vi "re_do_task_lua.vi"(5 "LuaVIEW reference":T1) -> (15 "error out":errorcluster)   [LabVIEW 2012]
doc: "Call the \"Do Task\" Lua API VI to prepare, pre-process, and execute a task script. Though this creates a seperate execution context, this function is synchronous because it waits for the task to finish.\n\nBy calling this function through <code>lv.pcall()</code>, you can execute, in a task context, a bit of code that can throw errors or has other ill-defined behaviour without risking the termination of your script or the corruption of its variable space.\n\nIf the task script is contained in a file, a relative path or bare filename will be resolved by searching relative to the configured script search directories. If no script search directories are configured, the resource base path is searched. If this function is called from a task context, the directory holding the main script of the calling task is searched first.\nParameters:\nstr:name, when the optional task script string is not specified, this is the filename plus any path from which to load the task script. Otherwise it is the name used to refer to the task script when reporting errors.\n[str:script], optional task script string allows direct specification of a bit of Lua code.\nErrors:\nCould not load task script or import script.\nError while preprrocessing task script or import script.\nCompilation error in task script or import script.\nTask identifier already in use.\nAny error thrown while executing the task."
uses:
  typedefs/t_LuaVIEW Reference.ctl
  subvis/private/LuaVIEW Pull (path).vi
  subvis/private/LuaVIEW Pull (string).vi
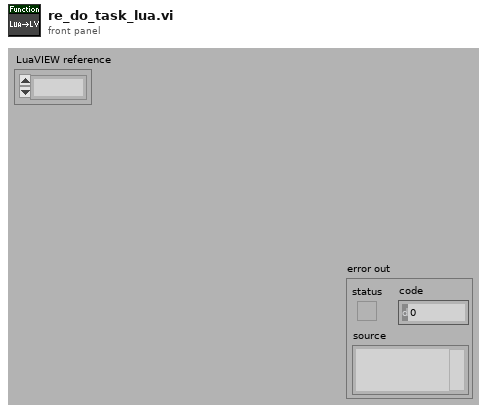
[diagram p1: front panel]
types:
  T1 = typedef "t_LuaVIEW Reference.ctl" = refnum<k1>
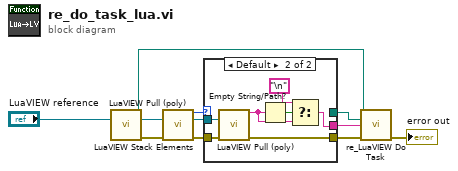
[diagram p0: block diagram]
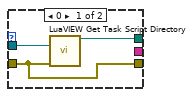
[diagram p2: hidden frame]
diagram:
  n1 = call-poly "LuaVIEW Pull (poly).vi"("LuaVIEW reference in"="LuaVIEW reference") -> ("path"=w1:path, "LuaVIEW reference out"=w9:T1, "error out"=w10:errorcluster)  [unwired: 12 in]
  n2 = call "LuaVIEW Stack Elements.vi"("LuaVIEW reference in"=w9, "error in (no error)"=w10) -> ("elements"=w8:i32, "LuaVIEW reference out"=w5:T1, "error out"=w7:errorcluster)  [unwired: 11 in]
  n3 = case shown="Default" w8 {
    tunnel: w7 -> [w14 w21]
    tunnel: [w14 w20] -> w3
    tunnel: [_ w19] -> w6
    tunnel: w5 -> [w12 w15]
    tunnel: [w13 _] -> w4
    frame 0 {
      n4 = call "LuaVIEW Get Task Script Directory.vi"("LuaVIEW reference in"=w12, "error in (no error)"=w14) -> ("task script directory"=w13:path)  [unwired: 11 in, 2 out]
    }
    frame Default {
      n5 = call-poly "LuaVIEW Pull (poly).vi"("LuaVIEW reference in"=w15, "error in (no error)"=w21) -> ("string"=w17:string, "error out"=w20:errorcluster)  [unwired: 11 in, 1 out]
      n6 = Empty String/Path?(string/path=w17) -> (empty?=w18:bool)
      n7 = Select(t="\n", s=w18, f=w17) -> (s? t:f=w19:string)
    }
  }
  n8 = call "re_LuaVIEW Do Task.vi"("script file or name (no name)"=w1, "custom search directory (none)"=w4, "script string (\"\" == load from file)"=w6, "error in (no error)"=w3) -> ("error out"=→"error out":errorcluster)  [unwired: 11 in]
